vi "Module Path.vi"(8 "error in (no error)":errorcluster) -> (0 "error out":errorcluster, 3 "Path":path)   [LabVIEW 2020, in "g_ar_toolkit.common.lvlib"]
uses:
  g_ar_toolkit.common.lvlib
  bin/g_ar_toolkit.1.32.dll
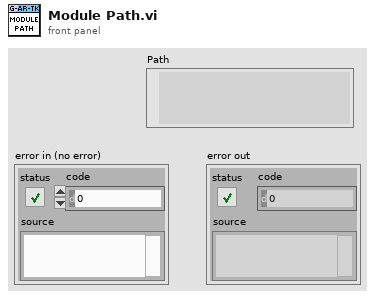
[diagram p1: front panel]
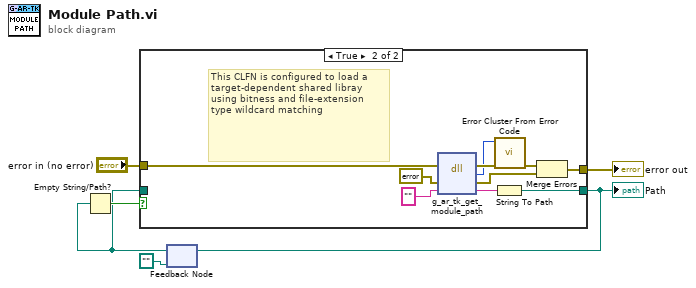
[diagram p0: block diagram]
diagram:
  n1 = feedback #1(path "") -> (w2:path)
  n2 = Empty String/Path?(string/path=w2) -> (empty?=w3:bool)
  n3 = case shown="True" w3 {
    tunnel: [w7 w12] -> w6
    tunnel: "error in (no error)" -> [w7 w11]
    tunnel: [w8 w9] -> w4
    tunnel: w2 -> [w8 _]
    frame False {
    }
    frame True {
      # "This CLFN is configured to load a target-dependent shared libray using bitness and file-extension type wildcard matching"
      n4 = dll-call lib="C:/serenial/libraries/g-augmented-reality-toolkit/LabVIEW/g_ar_toolkit.common/bin/g_ar_toolkit.1.*.*" fn="g_ar_tk_get_module_path" ("g_ar_toolkit.*.*:g_ar_tk_image_copy")(error in=w11, "error_cluster"=errorcluster {"status"=FALSE, "code"=0, "source"=""} ("error constant"), "path"="") -> (error out=w17:errorcluster, "MgErr"=w14:i32, "error_cluster"=w15:errorcluster, "path"=w10:string)  [unwired: 2 in, 1 out]
      n5 = String To Path(string=w10) -> (path=w9:path)
      n6 = call <vilib>:"Error Cluster From Error Code.vi"("error in (no error)"=w17, "error code (0)"=w14) -> ("error out"=w16:errorcluster)  [unwired: 7 in]
      n7 = Merge Errors(w16, w15) -> (w12:errorcluster)
    }
  }
  "error out" <- w6
  "Path" <- w4
  n8 = feedback-in #1(w4) -> ()
